vi "Compute Actor-Interface Status.vi"(10 "Array":T1[](array[typedef])) -> (1 "Any Message Out of Date?":bool, 2 "Actor/Interface Status":T1)   [LabVIEW 2023, in "Message Maker.lvclass"]
uses:
  Message Maker.lvclass
  Message Status.ctl
  Message Maker.lvclass/Message Maker.ctl
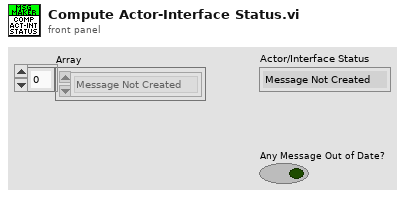
[diagram p1: front panel]
types:
  T1 = typedef "Message Maker.lvclass/Message Status.ctl" = enum16{"Message Not Created", "Message Out of Date", "Message OK", "Never update"}
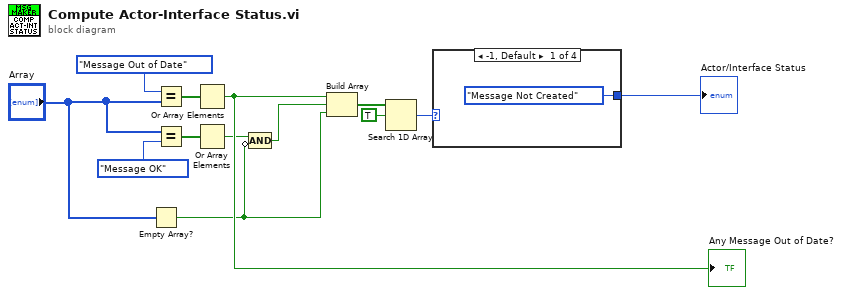
[diagram p0: block diagram]
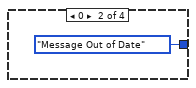
[diagram p2: hidden frame]
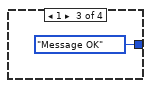
[diagram p3: hidden frame]
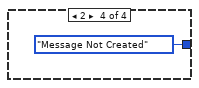
[diagram p4: hidden frame]
diagram:
  n1 = Empty Array?(array="Array") -> (empty?=w12:bool)
  n2 = Equal?(x=Message_Status."Message Out of Date" ("Message Status"), y="Array") -> (x = y?=w2:bool[])
  n3 = Equal?(x="Array", y=Message_Status."Message OK" ("Message Status")) -> (x = y?=w4:bool[])
  n4 = Or Array Elements(Boolean array=w2) -> (logical OR=w13:bool)
  "Any Message Out of Date?" <- w13
  n5 = Or Array Elements(Boolean array=w4) -> (logical OR=w10:bool)
  n6 = Compound Arithmetic op=AND(w10, invert w12) -> (w11:bool)
  n7 = Build Array(w13, w11, w12) -> (w5:bool[])
  n8 = Search 1D Array(1D array=w5, element=TRUE) -> (index of element=w7:i32)  [unwired: 1 in]
  n9 = case shown="-1, Default" w7 {
    tunnel: [Message_Status."Message Not Created" ("Message Status") Message_Status."Message Out of Date" ("Message Status") Message_Status."Message OK" ("Message Status") Message_Status."Message Not Created" ("Message Status")] -> w8
    frame -1, Default {
    }
    frame 0 {
    }
    frame 1 {
    }
    frame 2 {
    }
  }
  "Actor/Interface Status" <- w8
